vi "Read configuration.vi"(7 "force loading?":bool=TRUE, 8 "error in (no error)":errorcluster, 11 "focus in":refnum<class "focus.lvclass">) -> (0 "error out":errorcluster, 3 "focus out":refnum<class "focus.lvclass">)   [LabVIEW 2012]
doc: "Reads the XML-based configuration file and populates the configuration cluster accordingly. Configuration file name is <component ID>.xml."
uses:
  <vilib>/Distrio/Murmex/Murmex/Murmex.lvclass
  focus.lvclass
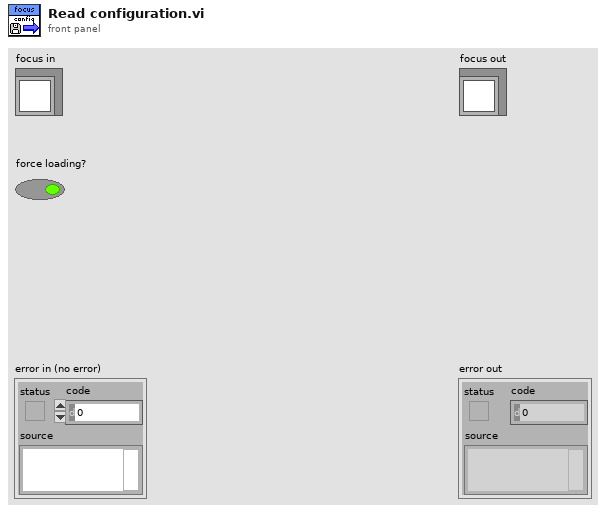
[diagram p1: front panel]
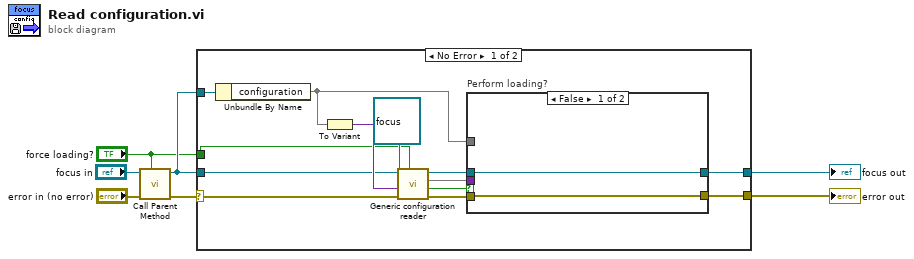
[diagram p0: block diagram]
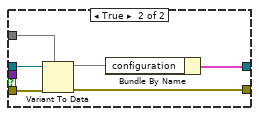
[diagram p2: hidden frame]
diagram:
  n1 = call-parent "Call Parent Method"("force loading?"="force loading?", "error in (no error)"="error in (no error)", "Murmex in"="focus in") -> ("error out"=w5:errorcluster, "Murmex out"=w4:refnum<class "focus.lvclass">)  [unwired: 7 in]
  n2 = case shown="No Error" w5 {
    selector: w5 -> [w18 w30]
    tunnel: w4 -> [w20 _]
    tunnel: w4 -> [w16 w31]
    tunnel: "force loading?" -> [w15 _]
    tunnel: [w9 w30] -> w2
    tunnel: [w8 w31] -> w1
    frame No Error {
      n3 = Unbundle By Name(w20) -> ("configuration"=w10)
      n4 = To Variant(anything=w10) -> (Variant=w19:variant)
      n5 = call <vilib>:"Generic configuration reader.vi"(7:w15, "error in (no error)"=w18, 9:w19, 10:refnum<class "focus.lvclass"> refnum ("focus"), "Murmex in"=w16) -> ("error out"=w14:errorcluster, "loaded?"=w12:bool, 2:w13, "Murmex out"=w11:refnum<class "focus.lvclass">)  [unwired: 3 in]
      n6 = case "Perform loading?" shown="False" w12 {
        tunnel: w10 -> [_ w29]
        tunnel: [w22 w27] -> w9
        tunnel: [w21 w26] -> w8
        tunnel: w14 -> [w22 w23]
        tunnel: w11 -> [w21 w25]
        tunnel: w13 -> [_ w24]
        frame False {
        }
        frame True {
          n7 = Variant To Data(error in=w23, type=w29, Variant=w24) -> (data=w28, error out=w27:errorcluster)
          n8 = Bundle By Name(cluster=w25, "configuration"=w28) -> (w26:cluster{})
        }
      }
    }
    frame Error {
    }
  }
  "error out" <- w2
  "focus out" <- w1
